vi "Get Input Parameters.vi"(8 "error in (no error)":errorcluster, 11 "Mock VI Call In":refnum<class "Mock VI Call.lvclass">) -> (0 "error out":errorcluster, 2 "Input Parameters":map{string, variant}(c390))   [LabVIEW 2020, in "Mock VI Call.lvclass"]
uses:
  Mock VI Call.lvclass
  Mock VI Call.lvclass/Mock VI Call.ctl
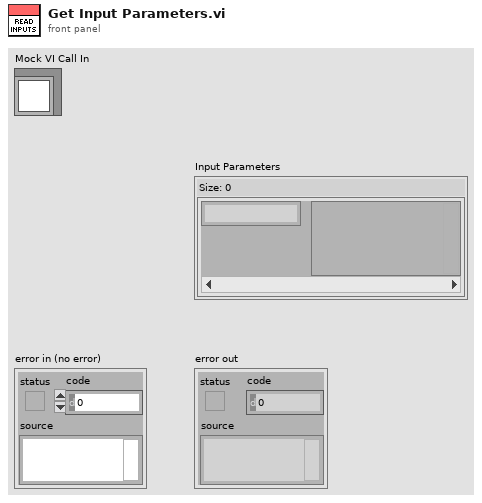
[diagram p1: front panel]
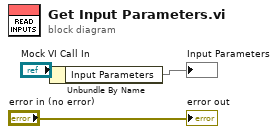
[diagram p0: block diagram]
diagram:
  n1 = Unbundle By Name("Mock VI Call In") -> ("Input Parameters"=→"Input Parameters":map{string, variant})
  "error out" <- "error in (no error)"
